vi "CalcAhWh.vi"(9 "I":dbl[](array[numeric]), 10 "V":dbl[](array[numeric]), 11 "T":dbl[](array[numeric])) -> ()   [LabVIEW 2025]
uses:
  Globals.vi
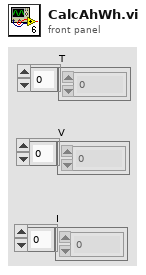
[diagram p1: front panel]
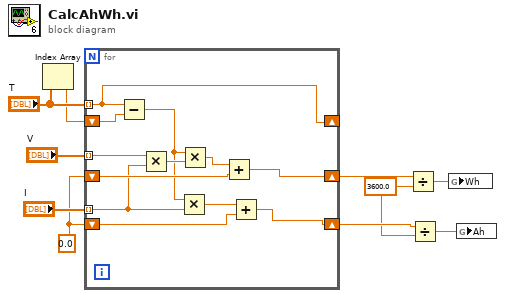
[diagram p0: block diagram]
diagram:
  w2 = 3600.0 ("y")
  w6 = 0.0
  n1 = Index Array(array="T") -> (element=w7:dbl)  [unwired: 1 in]
  n2 = for {
    tunnel: "T" -> [w21] mode=indexing
    tunnel: "V" -> [w20] mode=indexing
    tunnel: "I" -> [w14] mode=indexing
    shift-right: [w21] -> _
    shift-left: w7 -> [w22]
    shift-right: [w16] -> w5
    shift-left: w6 -> [w17]
    shift-right: [w11] -> w3
    shift-left: w6 -> [w12]
    n3 = Subtract(x=w21, y=w22) -> (x-y=w15:dbl)
    n4 = Multiply(x=w20, y=w14) -> (x*y=w19:dbl)
    n5 = Multiply(x=w15, y=w14) -> (x*y=w13:dbl)
    n6 = Multiply(x=w15, y=w19) -> (x*y=w18:dbl)
    n7 = Add(x=w18, y=w17) -> (x+y=w16:dbl)
    n8 = Add(x=w13, y=w12) -> (x+y=w11:dbl)
  }
  n9 = Divide(x=w5, y=w2) -> (x/y=w4:dbl)
  n10 = Divide(x=w3, y=w2) -> (x/y=w1:dbl)
  n11 = global write "Globals.vi" "Wh"(w4) -> ()
  n12 = global write "Globals.vi" "Ah"(w1) -> ()
